vi "TL2100LAB02.vi"() -> ()   [LabVIEW 2020]
panel:
  out "Inactive":bool
  out "FlowRate":dbl(slide) scale=-40000.0..40000.0
  out "Sensor Voltage":dbl
  out "SCC Volts":dbl format="%.3f"
  out "AtoD":i16 format="%04x"
  in  "Stop":bool
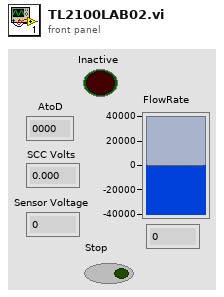
[diagram p1: front panel]
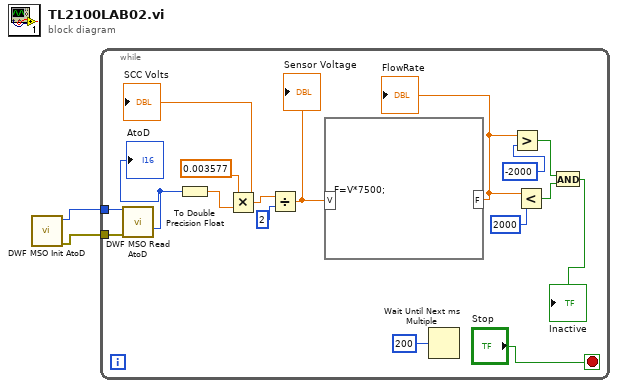
[diagram p0: block diagram]
diagram:
  n1 = call "DWF MSO Init AtoD.vi"() -> ("Error Out"=w1:errorcluster, "Instrument Handle Out"=w2:u32)  [unwired: 10 in]
  n2 = while {
    tunnel: w2 -> [w14]
    tunnel: w1 -> [w13]
    stop <- "Stop" stop-if-true
    n3 = call "DWF MSO Read AtoD.vi"("Instrument Handle In AtoD"=w14, "Error In"=w13) -> ("AtoD"=w12:i16)  [unwired: 12 in, 1 out]
    "AtoD" <- w12
    n4 = To Double Precision Float(number=w12) -> (double precision float=w16:dbl)
    n5 = Multiply(x=0.003577, y=w16) -> (x*y=w11:dbl)
    "SCC Volts" <- w11
    n6 = Divide(x=w11, y=2) -> (x/y=w9:dbl)
    "Sensor Voltage" <- w9
    n7 = formula code="F=V*7500;"("V"=w9) -> ("F"=w4:dbl)
    "FlowRate" <- w4
    n8 = Wait Until Next ms Multiple(millisecond multiple=200) -> ()  [unwired: 1 out]
    n9 = Greater?(x=w4, y=-2000) -> (0:w7:bool)
    n10 = Less?(x=w4, y=2000) -> (x < y?=w8:bool)
    n11 = And(x=w7, y=w8) -> (x .and. y?=→"Inactive":bool)
  }
